vi "Valves.vi"() -> ()   [LabVIEW 2013]
uses:
  SubVI/NI Modbus.llb/MB Serial Master Query Write Multiple Registers (poly).vi
  SubVI/NI Modbus.llb/MB Serial Master Query Write Multiple Coils (poly).vi
panel:
  in  "Serial Parameters":T1={"Mode"=enum."RTU", "Slave Address"=1}
  in  "Timeout":u32=10000
  in  "Flow Control":u16(ring) items=["None", "XON/XOFF", "RTS/CTS", "XON/XOFF & RTS/CTS", "DTR/DSR", "XON/XOFF & DTR/DSR"]
  in  "Parity":u16(ring) items=["None", "Odd", "Even", "Mark", "Space"]
  in  "Baud Rate":u32=9600
  in  "Port":refnum<visa-resource-name>
  in  "Stop":bool
  in  "Coils":bool[](array[boolean])=[FALSE, FALSE, FALSE, FALSE] caption="Coils to Write"
  in  "Registers":u16[](array[numeric])=[0, 0, 0, 0] caption="Registers to Write"
  # "Parametres"
  # "Valves"
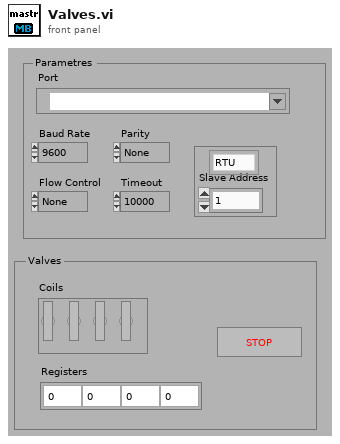
[diagram p1: front panel]
types:
  T1 = cluster{"Mode":enum16{"RTU", "ASCII"}, "Slave Address":u8}
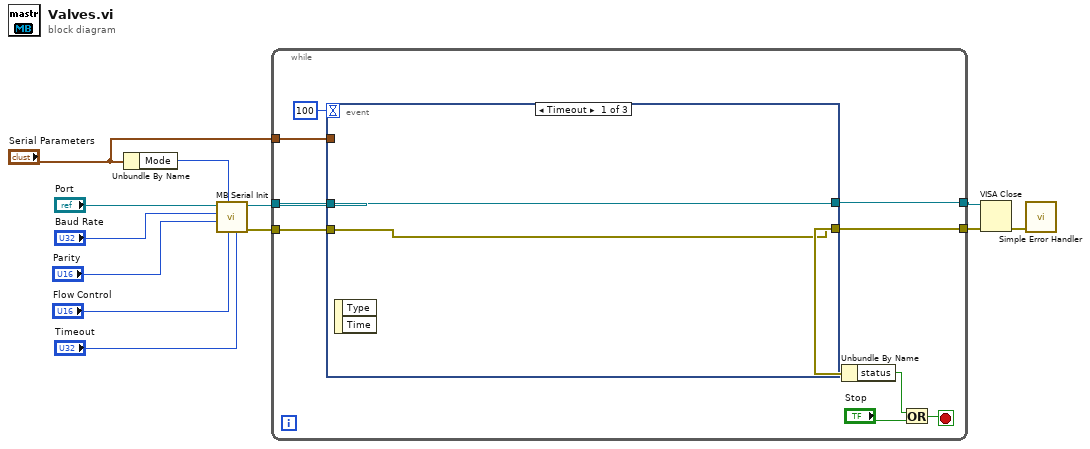
[diagram p0: block diagram]
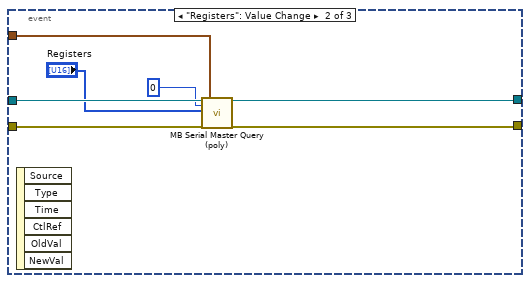
[diagram p2: hidden frame]
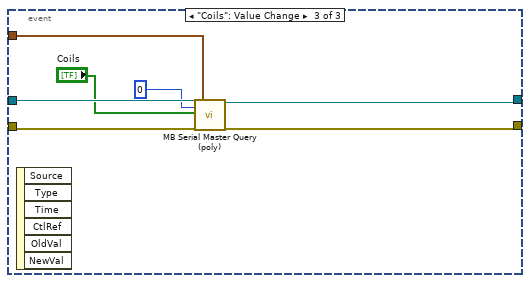
[diagram p3: hidden frame]
diagram:
  n1 = Unbundle By Name("Serial Parameters") -> ("Mode"=w6:enum16{"RTU", "ASCII"})
  n2 = call "MB Serial Init.vi"("Timeout"="Timeout", "Flow Control"="Flow Control", "Mode"=w6, "Parity"="Parity", "Baud Rate"="Baud Rate", "VISA resource name"="Port") -> ("error out"=w5:errorcluster, "VISA resource name out"=w11:refnum<visa-resource-name>)  [unwired: 1 in, 3 out]
  n3 = while {
    tunnel: w11 -> [w21]
    tunnel: w5 -> [w20]
    tunnel: "Serial Parameters" -> [w19]
    tunnel: [w15] -> w3
    tunnel: [w14] -> w2
    stop <- w18 stop-if-true
    n4 = event shown="[0] Timeout" {
      selector: _ -> [_ _ _]
      dyn-events: _ -> [_ _ _]
      timeout: 100 -> [_ _ _]
      tunnel: w21 -> [w23 w30 w37]
      tunnel: w20 -> [w22 w29 w36]
      tunnel: w19 -> [_ w28 w35]
      tunnel: [w22 w26 w31] -> w14
      tunnel: [w23 w25 w32] -> w15
      event Timeout {
        n5 = event-data() -> ()  [unwired: 3 out]
      }
      event "Registers": Value Change {
        n6 = event-data() -> ()  [unwired: 7 out]
        n7 = call-poly "MB Serial Master Query (poly).vi"("VISA resource name"=w30, "Starting Address"=u16 0, "Registers"="Registers", "error in"=w29, "Serial Parameters"=w28) -> ("VISA resource name out"=w25:refnum<visa-resource-name>, "error out"=w26:errorcluster)  [unwired: 2 in, 11 out]
      }
      event "Coils": Value Change {
        n8 = event-data() -> ()  [unwired: 7 out]
        n9 = call-poly "MB Serial Master Query (poly).vi"("VISA resource name"=w37, "Starting Address"=u16 0, "Coils"="Coils", "error in"=w36, "Serial Parameters"=w35) -> ("VISA resource name out"=w32:refnum<visa-resource-name>, "error out"=w31:errorcluster)  [unwired: 2 in, 11 out]
      }
    }
    n10 = Unbundle By Name(w14) -> ("status"=w16:bool)
    n11 = Or(x=w16, y="Stop") -> (x .or. y?=w18:bool)
  }
  n12 = VISA Close(VISA resource name=w3, error in (no error)=w2) -> (error out=w1:errorcluster)
  n13 = call <vilib>:"Simple Error Handler.vi"("error in (no error)"=w1) -> ()  [unwired: 1 in, 8 out]
